vi "host_main.vi"() -> ()   [LabVIEW 2023]
uses:
  JSON Command.ctl
  Action.ctl
  <vilib>/rvi/interface/nirviOpenFPGA/nirviOpenFPGA.xnode
  <vilib>/rvi/interface/nirviReadWriteControl/nirviReadWriteControl.xnode
  <vilib>/rvi/interface/nirviMethod/nirviMethod.xnode
  <vilib>/FPGAPlugInAG/Dynamic/niLvFpga_ConfigureFifo_Dynamic.vi
  <vilib>/rvi/errors/niLvFpgaMergeErrorWithErrorCode.vi
  <vilib>/FPGAPlugInAG/Dynamic/niLvFpga_Run_Dynamic.vi
  <vilib>/FPGAPlugInAG/Dynamic/niLvFpga_WriteFifo_Dynamic.vi
  NiFpgaLv.dll
  <vilib>/Utility/error.llb/Error Cluster From Error Code.vi
  <vilib>/rvi/interface/Simulation/niFpgaSimulationCallBeginRW.vi
  <vilib>/rvi/errors/niLvFpgaAdjustHostInterfaceError.vi
  <vilib>/rvi/interface/nirviCloseFPGA/nirviCloseFPGA.xnode
  <vilib>/FPGAPlugInAG/Dynamic/niLvFpga_ReadFifo_Dynamic.vi
  <vilib>/FPGAPlugInAG/Dynamic/niLvFpga_StopFifo_Dynamic.vi
  LabView workspace/CoboltLaserDriver.lvlib
  <vilib>/FPGAPlugInAG/Dynamic/niLvFpga_Close_Dynamic.vi
  FPGA Bitfiles/cryosimcontrolsy_FPGATarget_targetmainmem_OolXwFFypuY.lvbitx
  target_main_mem.vi
  <vilib>/FPGAPlugInAG/cRIO-9048/niLvFpga_Open_cRIO-9048.vi
  <vilib>/rvi/interface/common/dynamic/niFpgaDynamicAddResources.vi
panel:
  in  "Stop VI":bool
  out "FPGA VI Reference Out":refnum<k20>
  out "Abort":bool
  out "remote port":u16
  out "remote address":string
  in  "Send PORT":u16=7704
  out "From Client:":string
  out "RAW JSON":T1
  out "ACK sent":string
  in  "FPGA Status Update Loop Time (uSec)":u32=1000
  out "UDP Sent":string
  in  "Event":string
  in  "FPGA Status":string
  in  "Receive PORT":u16=7705
  in  "UDP Address (IP)":string="172.22.11.1"
  out "Digitals":u8
  out "Laser Response OK":bool=TRUE
  out "488 Blue Toggle":bool
  out "532 Red Toggle":bool
  out "638 Green Toggle":bool
  in  "Analogue Line 5":u32=20
  in  "Analogue Line 4":u32=20
  in  "Analogue Line 3":u32=20
  out "Analogue Line 2":u8
  out "Analogue Line 1":u8
  out "Analogue Line 0":u8
  out "Tick Ref":u32
  out "Addr Digitals":u32
  out "repDuration (ms)":u64
  out "numReps":u64
  out "From sendStartStopIndexes":u64[](array[numeric])
  out "Addr Analogue 1":u32
  out "Addr Analogue 2":u32
  out "Addr Analogue 0":u32
  in  "Digitals Action Table":T2[](array[typedef])
  in  "Analogue 2 Action Table":T2[](array[typedef])
  in  "Analogue 1 Action Table":T2[](array[typedef])
  in  "Analogue 0 Action Table":T2[](array[typedef])
  # "TCP Communication"
  # "UDP Communication"
  # "FPGA: Angle, Phase, and Color"
  # "FPGA: Laser On/Off and Power Control"
  # "Action Tables & Experiment Logging"
  # "Experiment Execution Trace"
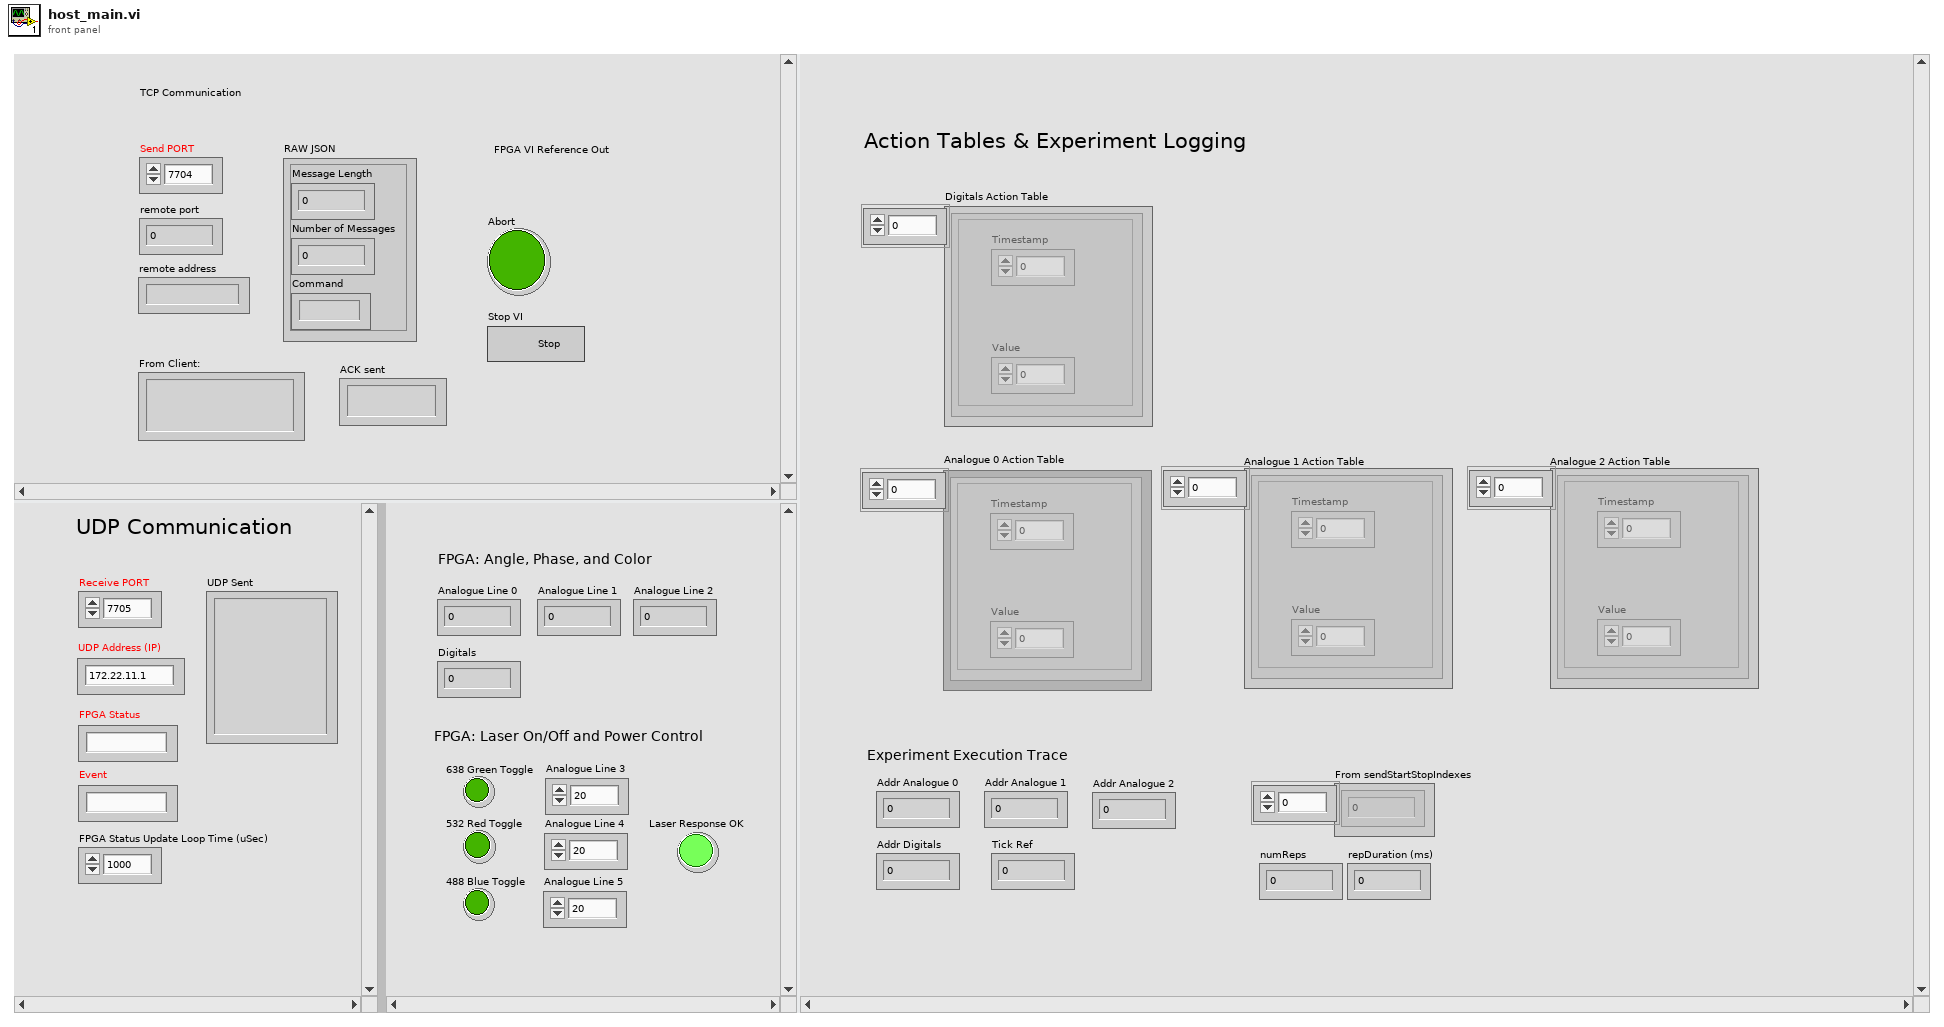
[diagram p1: front panel]
types:
  T1 = typedef "JSON Command.ctl" = cluster{"Message Length":i32, "Number of Messages":i32, "Command":string}
  T2 = typedef "Action.ctl" = cluster{"Timestamp":u32, "Value":u32}
  T3 = cluster{"Digital 0":bool, "Digital 1":bool, "Digital 2":bool}
  T4 = cluster{"Digitals":u8, "Analogue 0":u8, "Analogue 1":u8, "Event":string, "Analogue 2":u8, "Analogue 3":u32, "Analogue 4":u32, "Analogue 5":u32}
  T5 = enum16{"Standard", "Buffered", "CRLF", "Immediate"}
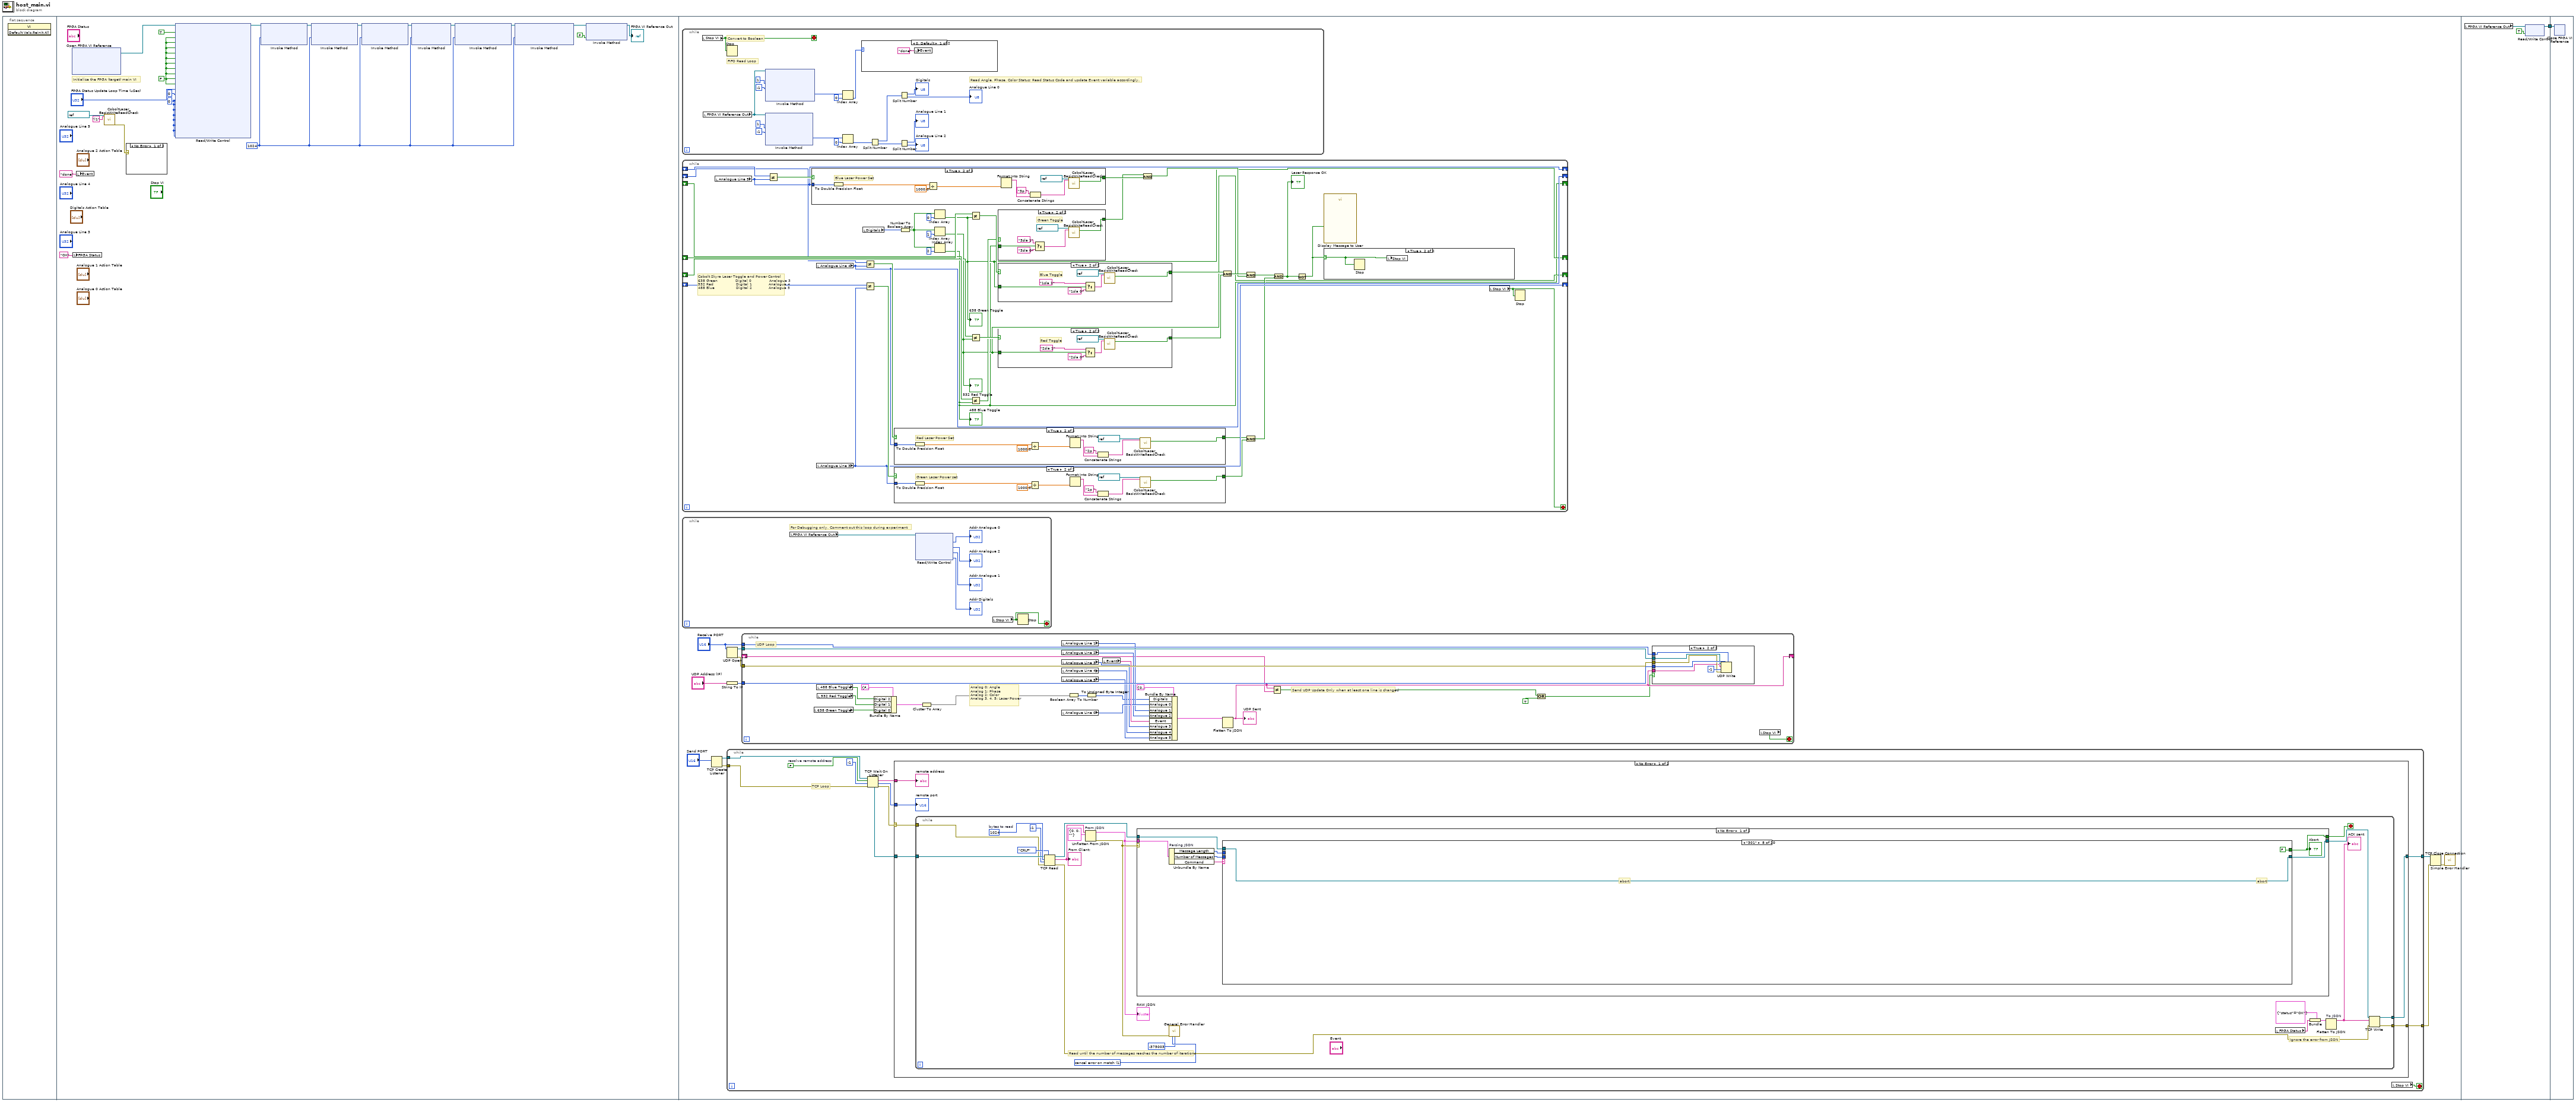
[diagram p0: block diagram]
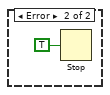
[diagram p2: hidden frame]
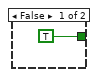
[diagram p4: hidden frame]
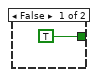
[diagram p5: hidden frame]
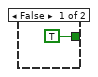
[diagram p6: hidden frame]
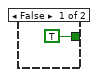
[diagram p7: hidden frame]
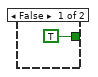
[diagram p8: hidden frame]
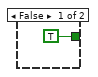
[diagram p9: hidden frame]
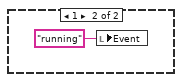
[diagram p10: hidden frame]
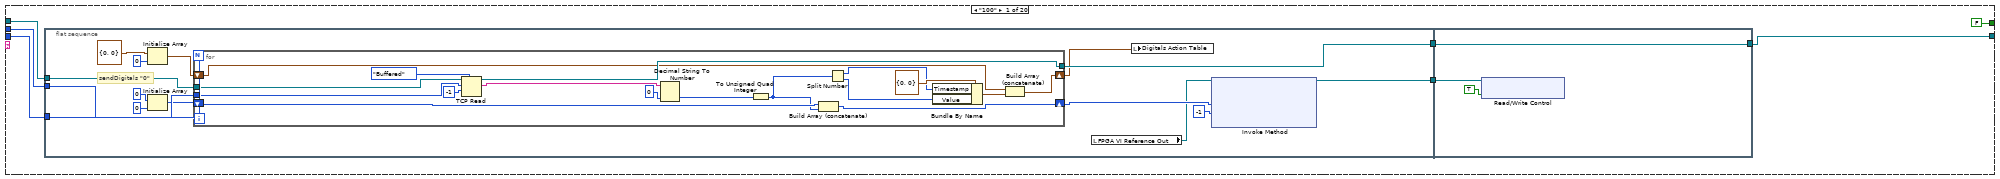
[diagram p12: hidden frame]
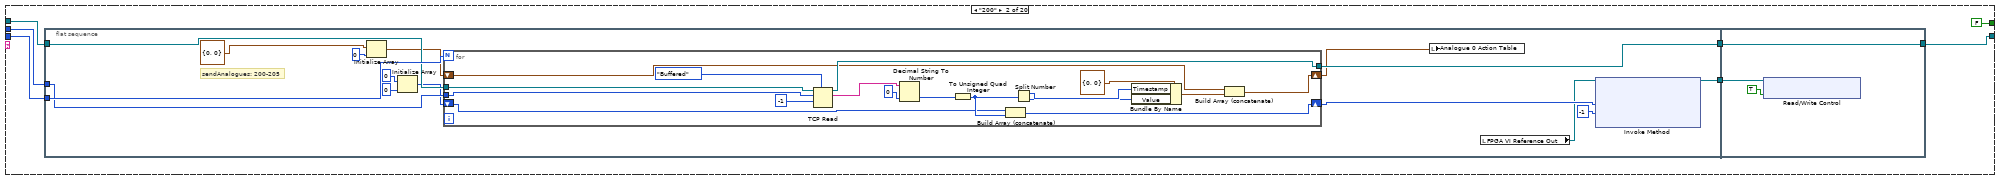
[diagram p13: hidden frame]
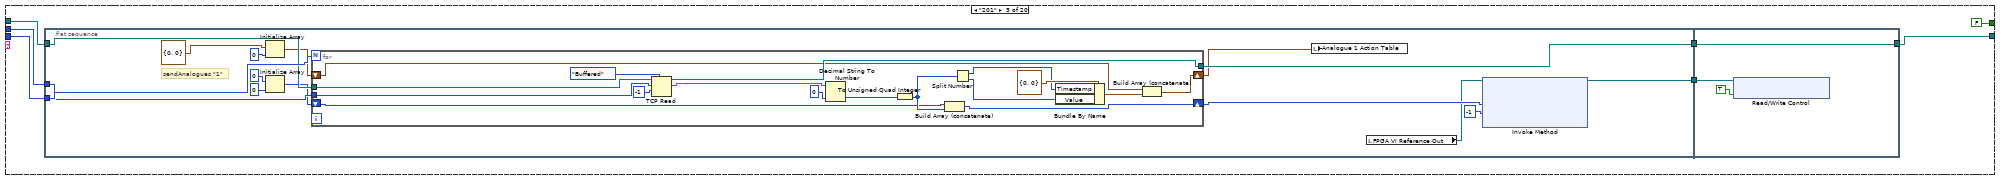
[diagram p14: hidden frame]
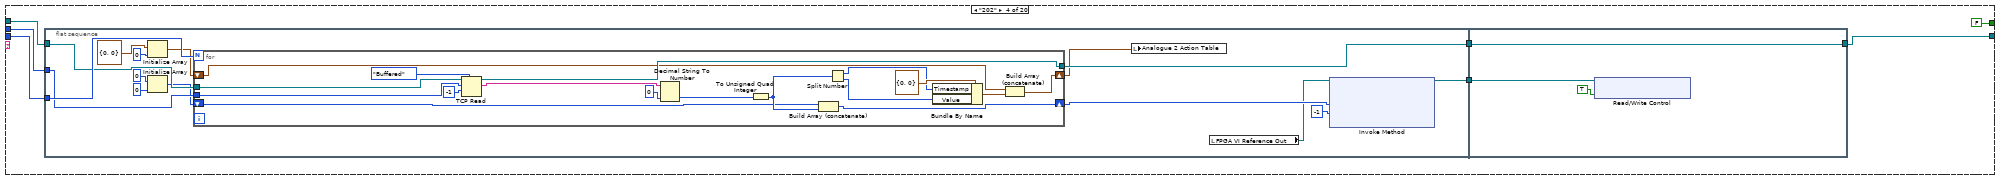
[diagram p15: hidden frame]
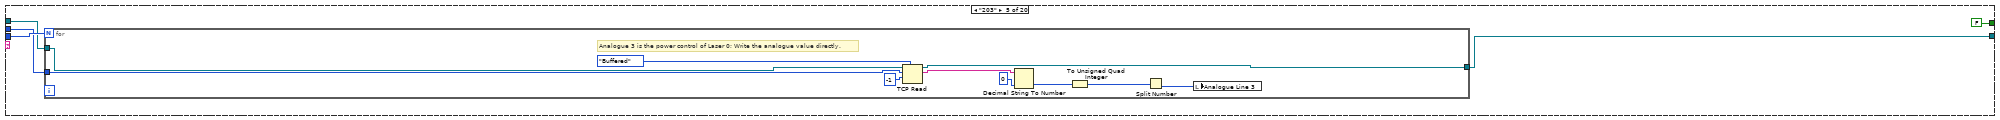
[diagram p16: hidden frame]
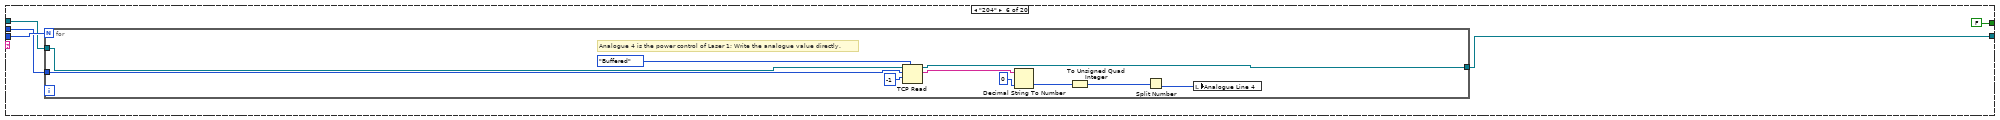
[diagram p17: hidden frame]
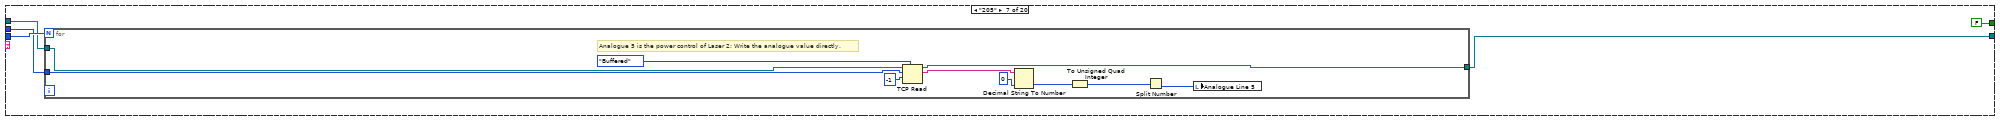
[diagram p18: hidden frame]
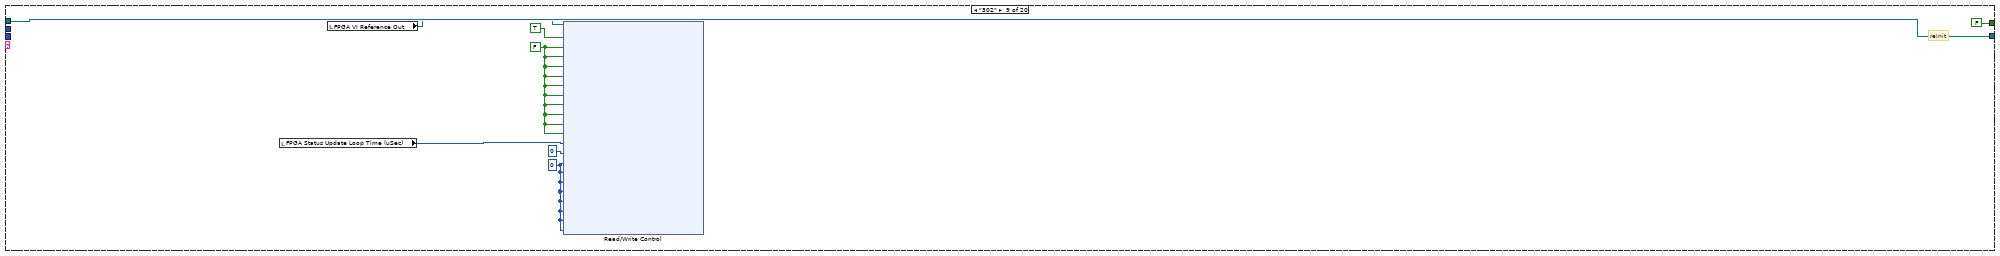
[diagram p19: hidden frame]
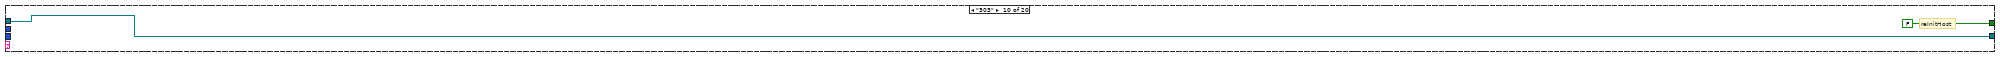
[diagram p20: hidden frame]
diagram:
  n1 = flat-sequence {
    tunnel: [w633] -> w1
    tunnel: w1 -> [w635]
    frame #0 {
      n2 = invoke class="VI" method="Default Vals.Reinit All"() -> ()  [unwired: 3 in, 3 out]
    }
    frame #1 {
      w5 = u32 0 ("Addr Analogue 0")
      w4 = u32 1024 ("Requested Depth")
      w2 = FALSE ("Action Abort")
      # "Initialize the FPGA (target) main VI"
      n3 = xnode "Open FPGA VI Reference"() -> ("FPGA VI Reference Out"=w11:refnum<k20>)  [unwired: 2 in, 1 out]
      n4 = local write "FPGA Status"("OK") -> ()
      n5 = local write "Event"("done") -> ()
      n6 = call "CoboltLaser_BasicWriteReadCheck.vi"("ComPort"=refnum<visa-resource-name> "COM4", "Command"="l1") -> ("error out"=w8:errorcluster)  [unwired: 22 in, 3 out]
      n7 = case shown="No Error" w8 {
        frame No Error {
        }
        frame Error {
          n8 = Stop(stop? (T)=TRUE) -> ()
        }
      }
      n9 = xnode "Read/Write Control"("FPGA VI Reference In"=w11, "FPGA Tick Reset"=TRUE, "Abort"=w2, "Load Actions Analogue 0"=w2, "Load Actions Analogue 1"=w2, "Load Actions Analogue 2"=w2, "Load Actions Digitals"=w2, "Flush FIFO"=w2, "Trigger Experiment"=w2, "Set Analogue 0"=w2, "Set Analogue 1"=w2, "Set Analogue 2"=w2, "FPGA Status Update Loop Time (uSec)"="FPGA Status Update Loop Time (uSec)", "Status Code"=u8 0, "Addr Analogue 0"=w5, "Addr Analogue 1"=w5, "Addr Analogue 2"=w5, "Num of Actions Analogue 0"=w5, "Num of Actions Analogue 1"=w5, "Num of Actions Analogue 2"=w5, "Num of Actions Digitals"=w5, "Digitals"=w5) -> ("FPGA VI Reference Out"=w7:refnum<k20>)  [unwired: 1 in, 1 out]
      n10 = xnode "Invoke Method"("FPGA VI Reference In"=w7, "Requested Depth"=w4) -> ("FPGA VI Reference Out"=w21:refnum<k20>)  [unwired: 1 in, 2 out]
      n11 = xnode "Invoke Method"("FPGA VI Reference In"=w21, "Requested Depth"=w4) -> ("FPGA VI Reference Out"=w12:refnum<k20>)  [unwired: 1 in, 2 out]
      n12 = xnode "Invoke Method"("FPGA VI Reference In"=w12, "Requested Depth"=w4) -> ("FPGA VI Reference Out"=w20:refnum<k20>)  [unwired: 1 in, 2 out]
      n13 = xnode "Invoke Method"("FPGA VI Reference In"=w20, "Requested Depth"=w4) -> ("FPGA VI Reference Out"=w19:refnum<k20>)  [unwired: 1 in, 2 out]
      n14 = xnode "Invoke Method"("FPGA VI Reference In"=w19, "Requested Depth"=w4) -> ("FPGA VI Reference Out"=w18:refnum<k20>)  [unwired: 1 in, 2 out]
      n15 = xnode "Invoke Method"("FPGA VI Reference In"=w18, "Requested Depth"=w4) -> ("FPGA VI Reference Out"=w6:refnum<k20>)  [unwired: 1 in, 2 out]
      n16 = xnode "Invoke Method"("FPGA VI Reference In"=w6, "Wait Until Done (F)"=FALSE) -> ("FPGA VI Reference Out"=→"FPGA VI Reference Out":refnum<k20>)  [unwired: 1 in, 1 out]
    }
    frame #2 {
      n17 = while {
        stop <- w130 stop-if-true
        # "Read Angle, Phase, Color Status; Read Status Code and update Event variable accordingly."
        # "FIFO Read Loop"
        # "Convert to Boolean"
        n18 = local read "Stop VI"() -> (w130:bool)
        n19 = local read "FPGA VI Reference Out"() -> (w131:refnum<k20>)
        n20 = Stop(stop? (T)=w130) -> ()
        n21 = xnode "Invoke Method"("FPGA VI Reference In"=w131, "Number of Elements"=u32 1, "Timeout (ms)"=-1) -> ("Data"=w135:u8[])  [unwired: 1 in, 3 out]
        n22 = xnode "Invoke Method"("FPGA VI Reference In"=w131, "Number of Elements"=u32 1, "Timeout (ms)"=-1) -> ("Data"=w144:u32[])  [unwired: 1 in, 3 out]
        n23 = Index Array(array=w135, index=0) -> (element=w136:u8)
        n24 = Index Array(array=w144, index=0) -> (element=w142:u32)
        n25 = case shown="0, Default" w136 {
          frame 0, Default {
            n26 = local write "Event"("done") -> ()
          }
          frame 1 {
            n27 = local write "Event"("running") -> ()
          }
        }
        n28 = Split Number(x=w142) -> (hi(x)=w141:u16, lo(x)=w140:u16)
        n29 = Split Number(x=w141) -> (hi(x)=→"Digitals":u8, lo(x)=→"Analogue Line 0":u8)
        n30 = Split Number(x=w140) -> (hi(x)=→"Analogue Line 1":u8, lo(x)=→"Analogue Line 2":u8)
      }
      n31 = while {
        shift-right: [w38] -> _
        shift-left: _ -> [w70]
        shift-right: [w36] -> _
        shift-left: _ -> [w65]
        shift-right: [w35] -> _
        shift-left: _ -> [w66]
        shift-right: [w58] -> _
        shift-left: _ -> [w61]
        shift-right: [w57] -> _
        shift-left: _ -> [w60]
        shift-right: [w56] -> _
        shift-left: _ -> [w59]
        stop <- w45 stop-if-true
        # "Cobolt Skyra Laser Toggle and Power Control\n638 Green               Digital 0               Analogue 3\n532 Red                   Digital 1              Analogue 4\n488 Blue                  Digital 2              Analogue 5"
        n32 = local read "Analogue Line 5"() -> (w58:u32)
        n33 = Not Equal?(x=w61, y=w58) -> (x != y?=w64:bool)
        n34 = case shown="True" w64 {
          tunnel: w58 -> [_ w96]
          tunnel: [TRUE w93] -> w53
          frame False {
          }
          frame True {
            # "Blue Laser Power Set"
            n35 = To Double Precision Float(number=w96) -> (double precision float=w97:dbl)
            n36 = Divide(x=w97, y=1000.0) -> (x/y=w101:dbl)
            n37 = Format Into String(w101) -> (resulting string=w100:string)  [unwired: 3 in, 1 out]
            n38 = Concatenate Strings("3p " ("string"), w100) -> (w95:string)
            n39 = call "CoboltLaser_BasicWriteReadCheck.vi"("ComPort"=refnum<visa-resource-name> "COM4", "Command"=w95) -> ("ResponseOK"=w93:bool)  [unwired: 22 in, 3 out]
          }
        }
        n40 = local read "Analogue Line 4"() -> (w57:u32)
        n41 = local read "Analogue Line 3"() -> (w56:u32)
        n42 = local read "Digitals"() -> (w37:u8)
        n43 = Not Equal?(x=w60, y=w57) -> (x != y?=w63:bool)
        n44 = Not Equal?(x=w59, y=w56) -> (x != y?=w62:bool)
        n45 = case shown="True" w63 {
          tunnel: w57 -> [_ w86]
          tunnel: [TRUE w84] -> w51
          frame False {
          }
          frame True {
            # "Red Laser Power Set"
            n46 = To Double Precision Float(number=w86) -> (double precision float=w87:dbl)
            n47 = Divide(x=w87, y=1000.0) -> (x/y=w91:dbl)
            n48 = Format Into String(w91) -> (resulting string=w90:string)  [unwired: 3 in, 1 out]
            n49 = Concatenate Strings("2p " ("string"), w90) -> (w83:string)
            n50 = call "CoboltLaser_BasicWriteReadCheck.vi"("ComPort"=refnum<visa-resource-name> "COM4", "Command"=w83) -> ("ResponseOK"=w84:bool)  [unwired: 22 in, 3 out]
          }
        }
        n51 = case shown="True" w62 {
          tunnel: w56 -> [_ w76]
          tunnel: [TRUE w74] -> w50
          frame False {
          }
          frame True {
            # "Green Laser Power set"
            n52 = To Double Precision Float(number=w76) -> (double precision float=w77:dbl)
            n53 = Divide(x=w77, y=1000.0) -> (x/y=w81:dbl)
            n54 = Format Into String(w81) -> (resulting string=w80:string)  [unwired: 3 in, 1 out]
            n55 = Concatenate Strings("1p " ("string"), w80) -> (w73:string)
            n56 = call "CoboltLaser_BasicWriteReadCheck.vi"("ComPort"=refnum<visa-resource-name> "COM4", "Command"=w73) -> ("ResponseOK"=w74:bool)  [unwired: 22 in, 3 out]
          }
        }
        n57 = Number To Boolean Array(number=w37) -> (Boolean array=w39:bool[])
        n58 = Index Array(array=w39, index=0) -> (element=w38:bool)
        "638 Green Toggle" <- w38
        n59 = Index Array(array=w39, index=1) -> (element=w36:bool)
        "532 Red Toggle" <- w36
        n60 = Index Array(array=w39, index=2) -> (element=w35:bool)
        "488 Blue Toggle" <- w35
        n61 = Not Equal?(x=w70, y=w38) -> (x != y?=w69:bool)
        n62 = Not Equal?(x=w65, y=w36) -> (x != y?=w68:bool)
        n63 = Not Equal?(x=w66, y=w35) -> (x != y?=w67:bool)
        n64 = case shown="True" w67 {
          tunnel: w35 -> [_ w105]
          tunnel: [TRUE w103] -> w52
          frame False {
          }
          frame True {
            # "Green Toggle"
            n65 = Select(t="3sla 1", s=w105, f="3sla 0") -> (s? t:f=w104:string)
            n66 = call "CoboltLaser_BasicWriteReadCheck.vi"("ComPort"=refnum<visa-resource-name> "COM4", "Command"=w104) -> ("ResponseOK"=w103:bool)  [unwired: 22 in, 3 out]
          }
        }
        n67 = case shown="True" w69 {
          tunnel: w38 -> [_ w120]
          tunnel: [TRUE w117] -> w55
          frame False {
          }
          frame True {
            # "Blue Toggle"
            n68 = Select(t="1sla 1", s=w120, f="1sla 0") -> (s? t:f=w118:string)
            n69 = call "CoboltLaser_BasicWriteReadCheck.vi"("ComPort"=refnum<visa-resource-name> "COM4", "Command"=w118) -> ("ResponseOK"=w117:bool)  [unwired: 22 in, 3 out]
          }
        }
        n70 = case shown="True" w68 {
          tunnel: w36 -> [_ w111]
          tunnel: [TRUE w110] -> w54
          frame False {
          }
          frame True {
            # "Red Toggle"
            n71 = Select(t="2sla 1", s=w111, f="2sla 0") -> (s? t:f=w112:string)
            n72 = call "CoboltLaser_BasicWriteReadCheck.vi"("ComPort"=refnum<visa-resource-name> "COM4", "Command"=w112) -> ("ResponseOK"=w110:bool)  [unwired: 22 in, 3 out]
          }
        }
        n73 = And(x=w52, y=w53) -> (x .and. y?=w48:bool)
        n74 = And(x=w55, y=w54) -> (x .and. y?=w49:bool)
        n75 = And(x=w49, y=w48) -> (x .and. y?=w46:bool)
        n76 = And(x=w51, y=w50) -> (x .and. y?=w47:bool)
        n77 = And(x=w46, y=w47) -> (x .and. y?=w44:bool)
        "Laser Response OK" <- w44
        n78 = Not(x=w44) -> (.not. x?=w43:bool)
        n79 = call "Display Message to User"("Enable"=w43) -> ()  [unwired: 9 in, 2 out]
        n80 = case shown="True" w43 {
          selector: w43 -> [_ w71]
          frame False {
          }
          frame True {
            n81 = Stop(stop? (T)=w71) -> ()
            n82 = local write "Stop VI"(w71) -> ()
          }
        }
        n83 = local read "Stop VI"() -> (w45:bool)
        n84 = Stop(stop? (T)=w45) -> ()
      }
      n85 = while {
        stop <- w124 stop-if-true
        # "For Debugging only. Comment out this loop during experiment"
        n86 = local read "FPGA VI Reference Out"() -> (w125:refnum<k20>)
        n87 = xnode "Read/Write Control"("FPGA VI Reference In"=w125) -> ("Addr Analogue 0"=→"Addr Analogue 0":u32, "Addr Analogue 2"=→"Addr Analogue 2":u32, "Addr Analogue 1"=→"Addr Analogue 1":u32, "Addr Digitals"=→"Addr Digitals":u32)  [unwired: 1 in, 2 out]
        n88 = local read "Stop VI"() -> (w124:bool)
        n89 = Stop(stop? (T)=w124) -> ()
      }
      n90 = TCP Create Listener(10:"Send PORT") -> (0:w32:errorcluster, 3:w31:refnum<k5>)  [unwired: 4 in, 1 out]
      n91 = UDP Open(11:"Receive PORT") -> (port=w26:refnum<k16>, 0:w28:errorcluster)  [unwired: 4 in, 1 out]
      n92 = String To IP(1:"UDP Address (IP)") -> (0:w25:u32)
      n93 = while {
        tunnel: w31 -> [w192]
        tunnel: w32 -> [w191]
        tunnel: [w190] -> w33
        tunnel: [w189] -> w34
        stop <- w182 stop-if-true
        w186 = FALSE  # resolve remote address
        # "TCP Loop"
        n94 = TCP Wait On Listener(8:w191, 9:-1 ("timeout ms (wait forever: -1)"), 10:w186, 11:w192) -> (0:w187:errorcluster, 1:w184:u16, 2:w185:string, 4:w183:refnum<k5>)  [unwired: 1 out]
        n95 = case shown="No Error" w187 {
          selector: w187 -> [w195 w630]
          tunnel: w183 -> [w198 w631]
          tunnel: [w197 w630] -> w190
          tunnel: [w196 w631] -> w189
          tunnel: w185 -> [w193 _]
          tunnel: w184 -> [w194 _]
          frame No Error {
            n96 = while {
              tunnel: w195 -> [w209]
              tunnel: [w211] -> w197
              tunnel: w198 -> [w212]
              tunnel: [w210] -> w196
              stop <- w203 stop-if-true
              w207 = 1 items=["no exception", "cancel error on match", "set error on match"] ("[exception action] (none:0)")
              w218 = 1024  # bytes to read
              # "Ignore the error from JSON"
              # "Read until the number of messages reaches the number of iterations"
              n97 = TCP Read(connection ID=w212, bytes to read=w218, error in (no error)=w209, 7:T5."CRLF" ("mode (standard)"), 9:-1 ("timeout ms (25000)")) -> (connection ID out=w201:refnum<k5>, data out=w215:string, error out=w219:errorcluster)
              "From Client:" <- w215
              n98 = Unflatten From JSON "From JSON"(JSON string=w215, type and defaults=T1 {"Message Length"=0, "Number of Messages"=0, "Command"=""} ("JSON Command")) -> (value=w204:T1, error out=w205:errorcluster)  [unwired: 5 in]
              "RAW JSON" <- w204
              n99 = case shown="No Error" w205 {
                tunnel: w204 -> [w226 _]
                tunnel: [w224 TRUE] -> w203
                tunnel: w201 -> [w222 w628]
                tunnel: [w221 w628] -> w200
                frame No Error {
                  n100 = Unbundle By Name "Parsing JSON"(w226) -> ("Message Length"=w220:i32, "Number of Messages"=w223:i32, "Command"=w225:string)
                  n101 = case shown="\"301\"" w225 {
                    tunnel: [FALSE FALSE FALSE FALSE FALSE FALSE FALSE FALSE FALSE FALSE FALSE FALSE FALSE FALSE FALSE FALSE FALSE FALSE FALSE TRUE] -> w224
                    tunnel: w223 -> [w232 w274 w317 w358 w398 w413 w428 _ _ _ _ _ w477 w500 _ _ _ _ _ _]
                    tunnel: w222 -> [w231 w273 w315 w357 w397 w412 w427 w440 w448 w450 w453 w469 w478 w502 w516 w535 w557 w572 w624 w627]
                    tunnel: [w230 w272 w314 w355 w395 w410 w425 w440 w448 w450 w453 w469 w471 w491 w516 w535 w556 w563 w624 w627] -> w221
                    tunnel: w220 -> [w229 w271 w313 w356 w396 w411 w426 _ _ _ _ _ w476 w501 _ _ w554 w568 _ _]
                    frame "100" {
                      n102 = flat-sequence {
                        tunnel: w232 -> [w248]
                        tunnel: w231 -> [w247]
                        tunnel: w229 -> [w245]
                        tunnel: [w246] -> w228
                        tunnel: [w234] -> w227
                        tunnel: [w268] -> w230
                        tunnel: w228 -> [w268]
                        tunnel: w227 -> [w267]
                        frame #0 {
                          # "sendDigitals \"0\""
                          n103 = Initialize Array(T2 {"Timestamp"=0, "Value"=0} ("Action"), 0 ("dimension size")) -> (w240:T2[])
                          n104 = Initialize Array(u64 0 ("element"), 0 ("dimension size")) -> (w239:u64[])
                          n105 = for {
                            N: w248 -> [_]
                            tunnel: w247 -> [w264]
                            tunnel: [w263] -> w246
                            tunnel: w245 -> [w262]
                            shift-right: [w250] -> w237
                            shift-left: w239 -> [w252]
                            shift-right: [w253] -> w238
                            shift-left: w240 -> [w255]
                            n106 = TCP Read(connection ID=w264, bytes to read=w262, 7:T5."Buffered" ("mode (standard)"), 9:-1 ("timeout ms (25000)")) -> (connection ID out=w263:refnum<k5>, data out=w259:string)  [unwired: 1 in, 1 out]
                            n107 = Decimal String To Number(string=w259, default (0L)=u64 0 ("default (0 I32)")) -> (number=w260:u64)  [unwired: 1 in, 1 out]
                            n108 = To Unsigned Quad Integer(1:w260) -> (0:w251:u64)
                            n109 = Build Array (concatenate)(w252, w251) -> (w250:u64[])
                            n110 = Split Number(x=w251) -> (hi(x)=w257:u32, lo(x)=w256:u32)
                            n111 = Bundle By Name(cluster=T2 {"Timestamp"=0, "Value"=0} ("Action"), "Timestamp"=w257, "Value"=w256) -> (w254:T2)
                            n112 = Build Array (concatenate)(w255, w254) -> (w253:T2[])
                          }
                          n113 = local read "FPGA VI Reference Out"() -> (w235:refnum<k20>)
                          n114 = local write "Digitals Action Table"(w238) -> ()
                          n115 = xnode "Invoke Method"("FPGA VI Reference In"=w235, "Data"=w237, "Timeout (ms)"=-1) -> ("FPGA VI Reference Out"=w234:refnum<k20>)  [unwired: 1 in, 2 out]
                        }
                        frame #1 {
                          n116 = xnode "Read/Write Control"("FPGA VI Reference In"=w267, "Load Actions Digitals"=TRUE ("Load Actions")) -> ()  [unwired: 1 in, 2 out]
                        }
                      }
                    }
                    frame "200" {
                      n117 = flat-sequence {
                        tunnel: w274 -> [w290]
                        tunnel: w273 -> [w289]
                        tunnel: w271 -> [w287]
                        tunnel: [w288] -> w270
                        tunnel: [w276] -> w269
                        tunnel: [w310] -> w272
                        tunnel: w270 -> [w310]
                        tunnel: w269 -> [w309]
                        frame #0 {
                          # "sendAnalogues: 200-205"
                          n118 = Initialize Array(T2 {"Timestamp"=0, "Value"=0} ("Action"), 0 ("dimension size")) -> (w284:T2[])
                          n119 = Initialize Array(u64 0 ("element"), 0 ("dimension size")) -> (w280:u64[])
                          n120 = for {
                            N: w290 -> [_]
                            tunnel: w289 -> [w306]
                            tunnel: [w304] -> w288
                            tunnel: w287 -> [w303]
                            shift-right: [w294] -> w283
                            shift-left: w284 -> [w299]
                            shift-right: [w291] -> w279
                            shift-left: w280 -> [w292]
                            n121 = TCP Read(connection ID=w306, bytes to read=w303, 7:T5."Buffered" ("mode (standard)"), 9:-1 ("timeout ms (25000)")) -> (connection ID out=w304:refnum<k5>, data out=w301:string)  [unwired: 1 in, 1 out]
                            n122 = Decimal String To Number(string=w301, default (0L)=u64 0) -> (number=w302:u64)  [unwired: 1 in, 1 out]
                            n123 = To Unsigned Quad Integer(1:w302) -> (0:w293:u64)
                            n124 = Build Array (concatenate)(w292, w293) -> (w291:u64[])
                            n125 = Split Number(x=w293) -> (hi(x)=w297:u32, lo(x)=w296:u32)
                            n126 = Bundle By Name(cluster=T2 {"Timestamp"=0, "Value"=0} ("Action"), "Timestamp"=w297, "Value"=w296) -> (w295:T2)
                            n127 = Build Array (concatenate)(w299, w295) -> (w294:T2[])
                          }
                          n128 = local write "Analogue 0 Action Table"(w283) -> ()
                          n129 = local read "FPGA VI Reference Out"() -> (w277:refnum<k20>)
                          n130 = xnode "Invoke Method"("FPGA VI Reference In"=w277, "Data"=w279, "Timeout (ms)"=-1) -> ("FPGA VI Reference Out"=w276:refnum<k20>)  [unwired: 1 in, 2 out]
                        }
                        frame #1 {
                          n131 = xnode "Read/Write Control"("FPGA VI Reference In"=w309, "Load Actions Analogue 0"=TRUE ("Load Actions")) -> ()  [unwired: 1 in, 2 out]
                        }
                      }
                    }
                    frame "201" {
                      n132 = flat-sequence {
                        tunnel: w317 -> [w332]
                        tunnel: w315 -> [w331]
                        tunnel: w313 -> [w329]
                        tunnel: [w330] -> w312
                        tunnel: [w318] -> w311
                        tunnel: [w352] -> w314
                        tunnel: w312 -> [w352]
                        tunnel: w311 -> [w351]
                        frame #0 {
                          # "sendAnalogues \"1\""
                          n133 = Initialize Array(T2 {"Timestamp"=0, "Value"=0} ("Action"), 0 ("dimension size")) -> (w326:T2[])
                          n134 = Initialize Array(u64 0, 0 ("dimension size")) -> (w321:u64[])
                          n135 = for {
                            N: w332 -> [_]
                            tunnel: w331 -> [w349]
                            tunnel: [w348] -> w330
                            tunnel: w329 -> [w347]
                            shift-right: [w338] -> w324
                            shift-left: w326 -> [w339]
                            shift-right: [w335] -> w320
                            shift-left: w321 -> [w336]
                            n136 = TCP Read(connection ID=w349, bytes to read=w347, 7:T5."Buffered" ("mode (standard)"), 9:-1 ("timeout ms (25000)")) -> (connection ID out=w348:refnum<k5>, data out=w344:string)  [unwired: 1 in, 1 out]
                            n137 = Decimal String To Number(string=w344, default (0L)=u64 0 ("default (0 I32)")) -> (number=w343:u64)  [unwired: 1 in, 1 out]
                            n138 = To Unsigned Quad Integer(1:w343) -> (0:w337:u64)
                            n139 = Build Array (concatenate)(w336, w337) -> (w335:u64[])
                            n140 = Split Number(x=w337) -> (hi(x)=w334:u32, lo(x)=w342:u32)
                            n141 = Bundle By Name(cluster=T2 {"Timestamp"=0, "Value"=0} ("Action"), "Timestamp"=w334, "Value"=w342) -> (w340:T2)
                            n142 = Build Array (concatenate)(w339, w340) -> (w338:T2[])
                          }
                          n143 = local write "Analogue 1 Action Table"(w324) -> ()
                          n144 = local read "FPGA VI Reference Out"() -> (w319:refnum<k20>)
                          n145 = xnode "Invoke Method"("FPGA VI Reference In"=w319, "Data"=w320, "Timeout (ms)"=-1) -> ("FPGA VI Reference Out"=w318:refnum<k20>)  [unwired: 1 in, 2 out]
                        }
                        frame #1 {
                          n146 = xnode "Read/Write Control"("FPGA VI Reference In"=w351, "Load Actions Analogue 1"=TRUE ("Load Actions")) -> ()  [unwired: 1 in, 2 out]
                        }
                      }
                    }
                    frame "202" {
                      n147 = flat-sequence {
                        tunnel: w358 -> [w374]
                        tunnel: w357 -> [w369]
                        tunnel: w356 -> [w368]
                        tunnel: [w367] -> w354
                        tunnel: [w361] -> w353
                        tunnel: [w394] -> w355
                        tunnel: w354 -> [w394]
                        tunnel: w353 -> [w393]
                        frame #0 {
                          n148 = Initialize Array(T2 {"Timestamp"=0, "Value"=0} ("Action"), 0 ("dimension size")) -> (w366:T2[])
                          n149 = Initialize Array(u64 0 ("element"), 0 ("dimension size")) -> (w364:u64[])
                          n150 = for {
                            N: w374 -> [_]
                            tunnel: w369 -> [w390]
                            tunnel: w368 -> [w389]
                            tunnel: [w386] -> w367
                            shift-right: [w379] -> w365
                            shift-left: w366 -> [w380]
                            shift-right: [w376] -> w363
                            shift-left: w364 -> [w377]
                            n151 = TCP Read(connection ID=w390, bytes to read=w389, 7:T5."Buffered" ("mode (standard)"), 9:-1 ("timeout ms (25000)")) -> (connection ID out=w386:refnum<k5>, data out=w387:string)  [unwired: 1 in, 1 out]
                            n152 = Decimal String To Number(string=w387, default (0L)=u64 0 ("default (0 I32)")) -> (number=w385:u64)  [unwired: 1 in, 1 out]
                            n153 = To Unsigned Quad Integer(1:w385) -> (0:w378:u64)
                            n154 = Build Array (concatenate)(w377, w378) -> (w376:u64[])
                            n155 = Split Number(x=w378) -> (hi(x)=w383:u32, lo(x)=w382:u32)
                            n156 = Bundle By Name(cluster=T2 {"Timestamp"=0, "Value"=0} ("Action"), "Timestamp"=w383, "Value"=w382) -> (w381:T2)
                            n157 = Build Array (concatenate)(w380, w381) -> (w379:T2[])
                          }
                          n158 = local write "Analogue 2 Action Table"(w365) -> ()
                          n159 = local read "FPGA VI Reference Out"() -> (w360:refnum<k20>)
                          n160 = xnode "Invoke Method"("FPGA VI Reference In"=w360, "Data"=w363, "Timeout (ms)"=-1) -> ("FPGA VI Reference Out"=w361:refnum<k20>)  [unwired: 1 in, 2 out]
                        }
                        frame #1 {
                          n161 = xnode "Read/Write Control"("FPGA VI Reference In"=w393, "Load Actions Analogue 2"=TRUE ("Load Actions")) -> ()  [unwired: 1 in, 2 out]
                        }
                      }
                    }
                    frame "203" {
                      n162 = for {
                        N: w398 -> [_]
                        tunnel: w397 -> [w408]
                        tunnel: w396 -> [w407]
                        tunnel: [w404] -> w395
                        # "Analogue 3 is the power control of Laser 0; Write the analogue value directly."
                        n163 = TCP Read(connection ID=w408, bytes to read=w407, 7:T5."Buffered" ("mode (standard)"), 9:-1 ("timeout ms (25000)")) -> (connection ID out=w404:refnum<k5>, data out=w405:string)  [unwired: 1 in, 1 out]
                        n164 = Decimal String To Number(string=w405, default (0L)=u64 0 ("default (0 I32)")) -> (number=w403:u64)  [unwired: 1 in, 1 out]
                        n165 = To Unsigned Quad Integer(1:w403) -> (0:w402:u64)
                        n166 = Split Number(x=w402) -> (lo(x)=w400:u32)  [unwired: 1 out]
                        n167 = local write "Analogue Line 3"(w400) -> ()
                      }
                    }
                    frame "204" {
                      n168 = for {
                        N: w413 -> [_]
                        tunnel: w412 -> [w423]
                        tunnel: w411 -> [w422]
                        tunnel: [w419] -> w410
                        # "Analogue 4 is the power control of Laser 1; Write the analogue value directly."
                        n169 = TCP Read(connection ID=w423, bytes to read=w422, 7:T5."Buffered" ("mode (standard)"), 9:-1 ("timeout ms (25000)")) -> (connection ID out=w419:refnum<k5>, data out=w420:string)  [unwired: 1 in, 1 out]
                        n170 = Decimal String To Number(string=w420, default (0L)=u64 0 ("default (0 I32)")) -> (number=w418:u64)  [unwired: 1 in, 1 out]
                        n171 = To Unsigned Quad Integer(1:w418) -> (0:w417:u64)
                        n172 = Split Number(x=w417) -> (lo(x)=w415:u32)  [unwired: 1 out]
                        n173 = local write "Analogue Line 4"(w415) -> ()
                      }
                    }
                    frame "205" {
                      n174 = for {
                        N: w428 -> [_]
                        tunnel: w427 -> [w438]
                        tunnel: w426 -> [w437]
                        tunnel: [w434] -> w425
                        # "Analogue 5 is the power control of Laser 2; Write the analogue value directly."
                        n175 = TCP Read(connection ID=w438, bytes to read=w437, 7:T5."Buffered" ("mode (standard)"), 9:-1 ("timeout ms (25000)")) -> (connection ID out=w434:refnum<k5>, data out=w435:string)  [unwired: 1 in, 1 out]
                        n176 = Decimal String To Number(string=w435, default (0L)=u64 0 ("default (0 I32)")) -> (number=w433:u64)  [unwired: 1 in, 1 out]
                        n177 = To Unsigned Quad Integer(1:w433) -> (0:w432:u64)
                        n178 = Split Number(x=w432) -> (lo(x)=w430:u32)  [unwired: 1 out]
                        n179 = local write "Analogue Line 5"(w430) -> ()
                      }
                    }
                    frame "301" {
                      # "abort"
                      # "abort"
                    }
                    frame "302" {
                      w445 = u32 0 ("Addr Analogue 0")
                      w444 = FALSE ("Action Abort")
                      # "reInit"
                      n180 = local read "FPGA Status Update Loop Time (uSec)"() -> (w442:u32)
                      n181 = local read "FPGA VI Reference Out"() -> (w443:refnum<k20>)
                      n182 = xnode "Read/Write Control"("FPGA VI Reference In"=w443, "FPGA Tick Reset"=TRUE, "Abort"=w444, "Load Actions Analogue 0"=w444, "Load Actions Analogue 1"=w444, "Load Actions Analogue 2"=w444, "Load Actions Digitals"=w444, "Flush FIFO"=w444, "Trigger Experiment"=w444, "Set Analogue 0"=w444, "Set Analogue 1"=w444, "Set Analogue 2"=w444, "FPGA Status Update Loop Time (uSec)"=w442, "Status Code"=u8 0, "Addr Analogue 0"=w445, "Addr Analogue 1"=w445, "Addr Analogue 2"=w445, "Num of Actions Analogue 0"=w445, "Num of Actions Analogue 1"=w445, "Num of Actions Analogue 2"=w445, "Num of Actions Digitals"=w445, "Digitals"=w445) -> ()  [unwired: 1 in, 2 out]
                    }
                    frame "303" {
                      # "reInitHost"
                    }
                    frame "304" {
                      # "reInitFPGA"
                      n183 = flat-sequence {
                        tunnel: [w458] -> w452
                        tunnel: w452 -> [w465]
                        frame #0 {
                          w457 = u32 0 ("Addr Analogue 0")
                          w455 = FALSE ("Abort")
                          w456 = TRUE ("FPGA Tick Reset")
                          n184 = local read "FPGA VI Reference Out"() -> (w464:refnum<k20>)
                          n185 = xnode "Read/Write Control"("FPGA VI Reference In"=w464, "FPGA Tick Reset"=w456, "Flush FIFO"=w456, "Load Actions Analogue 0"=w455, "Load Actions Analogue 1"=w455, "Load Actions Analogue 2"=w455, "Load Actions Digitals"=w455, "Abort"=w455, "Set Analogue 0"=w455, "Set Analogue 1"=w455, "Set Analogue 2"=w455, "Trigger Experiment"=w455, "Status Code"=u8 0, "Addr Analogue 0"=w457, "Addr Analogue 1"=w457, "Addr Analogue 2"=w457, "Addr Digitals"=w457, "Num of Actions Digitals"=w457, "Num of Actions Analogue 0"=w457, "Num of Actions Analogue 1"=w457, "Num of Actions Analogue 2"=w457) -> ("FPGA VI Reference Out"=w459:refnum<k20>)  [unwired: 1 in, 1 out]
                          n186 = xnode "Invoke Method"("FPGA VI Reference In"=w459) -> ("FPGA VI Reference Out"=w462:refnum<k20>)  [unwired: 1 in, 1 out]
                          n187 = xnode "Invoke Method"("FPGA VI Reference In"=w462) -> ("FPGA VI Reference Out"=w461:refnum<k20>)  [unwired: 1 in, 1 out]
                          n188 = xnode "Invoke Method"("FPGA VI Reference In"=w461) -> ("FPGA VI Reference Out"=w460:refnum<k20>)  [unwired: 1 in, 1 out]
                          n189 = xnode "Invoke Method"("FPGA VI Reference In"=w460) -> ("FPGA VI Reference Out"=w458:refnum<k20>)  [unwired: 1 in, 1 out]
                        }
                        frame #1 {
                          n190 = while {
                            tunnel: w465 -> [w466]
                            stop <- w467 stop-if-true
                            n191 = xnode "Read/Write Control"("FPGA VI Reference In"=w466) -> ("Flush FIFO"=w468:bool)  [unwired: 1 in, 2 out]
                            n192 = Not(x=w468) -> (.not. x?=w467:bool)
                          }
                        }
                      }
                    }
                    frame "405" {
                      # "updateNrReps"
                    }
                    frame "406" {
                      # "sendStartStopIndexes"
                      n193 = Initialize Array(u64 0 ("element"), 0 ("dimension size")) -> (w473:u64[])
                      n194 = for {
                        N: w477 -> [_]
                        tunnel: w478 -> [w489]
                        tunnel: w476 -> [w488]
                        shift-right: [w481] -> w472
                        shift-left: w473 -> [w484]
                        tunnel: [w480] -> w471
                        n195 = TCP Read(connection ID=w489, bytes to read=w488, 7:T5."Buffered" ("mode (standard)"), 9:-1 ("timeout ms (25000)")) -> (connection ID out=w480:refnum<k5>, data out=w486:string)  [unwired: 1 in, 1 out]
                        n196 = Decimal String To Number(string=w486, default (0L)=u64 0 ("default (0 I32)")) -> (number=w483:u64)  [unwired: 1 in, 1 out]
                        n197 = To Unsigned Quad Integer(1:w483) -> (0:w482:u64)
                        n198 = Build Array (concatenate)(w484, w482) -> (w481:u64[])
                      }
                      "From sendStartStopIndexes" <- w472
                    }
                    frame "407" {
                      # "initProfile"
                      n199 = Initialize Array(u64 0 ("element"), 0 ("dimension size")) -> (w497:u64[])
                      n200 = for {
                        N: w500 -> [_]
                        tunnel: w502 -> [w513]
                        tunnel: w501 -> [w512]
                        shift-right: [w505] -> w496
                        shift-left: w497 -> [w507]
                        tunnel: [w504] -> w491
                        n201 = TCP Read(connection ID=w513, bytes to read=w512, 9:-1 ("timeout ms (25000)")) -> (connection ID out=w504:refnum<k5>, data out=w510:string)  [unwired: 2 in, 1 out]
                        n202 = Decimal String To Number(string=w510, default (0L)=u64 0 ("default (0 I32)")) -> (number=w508:u64)  [unwired: 1 in, 1 out]
                        n203 = To Unsigned Quad Integer(1:w508) -> (0:w506:u64)
                        n204 = Build Array (concatenate)(w507, w506) -> (w505:u64[])
                      }
                      n205 = Index Array(array=w496, index=1) -> (element=→"repDuration (ms)":u64)
                      n206 = Index Array(array=w496, index=0) -> (element=→"numReps":u64)
                    }
                    frame "408" {
                      # "triggerExperiment"
                      n207 = local read "FPGA VI Reference Out"() -> (w515:refnum<k20>)
                      n208 = flat-sequence {
                        tunnel: w515 -> [w518]
                        tunnel: [w520] -> w514
                        tunnel: w514 -> [w533]
                        frame #0 {
                          n209 = while {
                            tunnel: w518 -> [w529]
                            stop <- w528 stop-if-true
                            # "wait until all actions loaded"
                            n210 = xnode "Read/Write Control"("FPGA VI Reference In"=w529) -> ("Load Actions Analogue 0"=w524:bool, "Load Actions Analogue 1"=w523:bool, "Load Actions Analogue 2"=w522:bool, "Load Actions Analogue 2"=w521:bool)  [unwired: 1 in, 2 out]
                            n211 = Or(x=w524, y=w523) -> (x .or. y?=w526:bool)
                            n212 = Or(x=w522, y=w521) -> (x .or. y?=w525:bool)
                            n213 = Or(x=w526, y=w525) -> (x .or. y?=w527:bool)
                            n214 = Not(x=w527) -> (.not. x?=w528:bool)
                          }
                          n215 = xnode "Read/Write Control"("FPGA VI Reference In"=w518, "FPGA Tick Reset"=TRUE) -> ("FPGA VI Reference Out"=w520:refnum<k20>)  [unwired: 1 in, 1 out]
                        }
                        frame #1 {
                          n216 = xnode "Read/Write Control"("FPGA VI Reference In"=w533, "FPGA Tick Reset"=FALSE, "Trigger Experiment"=TRUE ("FPGA Tick Reset")) -> ("Tick Ref"=→"Tick Ref":u32)  [unwired: 1 in, 2 out]
                        }
                      }
                    }
                    frame "409" {
                      # "flushFIFOs"
                      n217 = flat-sequence {
                        tunnel: [w538] -> w534
                        tunnel: w534 -> [w545]
                        frame #0 {
                          w537 = FALSE ("Load Actions")
                          n218 = local read "FPGA VI Reference Out"() -> (w544:refnum<k20>)
                          n219 = xnode "Read/Write Control"("FPGA VI Reference In"=w544, "Flush FIFO"=TRUE, "Load Actions Analogue 0"=w537, "Load Actions Analogue 1"=w537, "Load Actions Analogue 2"=w537, "Load Actions Digitals"=w537, "Set Analogue 0"=w537, "Set Analogue 1"=w537, "Set Analogue 2"=w537) -> ("FPGA VI Reference Out"=w542:refnum<k20>)  [unwired: 1 in, 1 out]
                          n220 = xnode "Invoke Method"("FPGA VI Reference In"=w542) -> ("FPGA VI Reference Out"=w541:refnum<k20>)  [unwired: 1 in, 1 out]
                          n221 = xnode "Invoke Method"("FPGA VI Reference In"=w541) -> ("FPGA VI Reference Out"=w540:refnum<k20>)  [unwired: 1 in, 1 out]
                          n222 = xnode "Invoke Method"("FPGA VI Reference In"=w540) -> ("FPGA VI Reference Out"=w539:refnum<k20>)  [unwired: 1 in, 1 out]
                          n223 = xnode "Invoke Method"("FPGA VI Reference In"=w539) -> ("FPGA VI Reference Out"=w538:refnum<k20>)  [unwired: 1 in, 1 out]
                        }
                        frame #1 {
                          n224 = while {
                            tunnel: w545 -> [w546]
                            stop <- w547 stop-if-true
                            # "wait until FPGA target flushes FIFO"
                            n225 = xnode "Read/Write Control"("FPGA VI Reference In"=w546) -> ("Flush FIFO"=w548:bool)  [unwired: 1 in, 2 out]
                            n226 = Not(x=w548) -> (.not. x?=w547:bool)
                          }
                        }
                      }
                    }
                    frame "410" {
                      # "writeDigitals"
                      n227 = TCP Read(connection ID=w557, bytes to read=w554, 7:T5."Buffered" ("mode (standard)"), 9:-1 ("timeout ms (25000)")) -> (connection ID out=w556:refnum<k5>, data out=w551:string)  [unwired: 1 in, 1 out]
                      n228 = local read "FPGA VI Reference Out"() -> (w550:refnum<k20>)
                      n229 = Decimal String To Number(string=w551, default (0L)=u32 0 ("default (0 I32)")) -> (number=w549:u32)  [unwired: 1 in, 1 out]
                      n230 = xnode "Read/Write Control"("FPGA VI Reference In"=w550, "Digitals"=w549) -> ()  [unwired: 1 in, 2 out]
                    }
                    frame "411" {
                      # "writeAnalogue"
                      n231 = TCP Read(connection ID=w572, bytes to read=w568, 7:T5."Buffered" ("mode (standard)"), 9:-1 ("timeout ms (25000)")) -> (connection ID out=w569:refnum<k5>, data out=w574:string, error out=w566:errorcluster)  [unwired: 1 in]
                      n232 = Decimal String To Number(string=w574, default (0L)=u32 0 ("default (0 I32)")) -> (number=w562:u32)  [unwired: 1 in, 1 out]
                      n233 = TCP Read(connection ID=w569, bytes to read=w568, error in (no error)=w566, 7:T5."Buffered" ("mode (standard)"), 9:-1 ("timeout ms (25000)")) -> (connection ID out=w563:refnum<k5>, data out=w564:string)  [unwired: 1 out]
                      n234 = local read "FPGA VI Reference Out"() -> (w559:refnum<k20>)
                      n235 = Decimal String To Number(string=w564, default (0L)=u32 0 ("default (0 I32)")) -> (number=w560:u32)  [unwired: 1 in, 1 out]
                      n236 = case shown="2" w562 {
                        tunnel: w560 -> [w578 w593 w608 w621 w622 w623 _]
                        tunnel: w559 -> [w579 w594 w609 _ _ _ _]
                        frame 0 {
                          n237 = flat-sequence {
                            tunnel: w579 -> [w584]
                            tunnel: w578 -> [w583]
                            tunnel: [w581] -> w577
                            tunnel: [w580] -> w576
                            tunnel: w577 -> [w586]
                            tunnel: w576 -> [w585]
                            frame #0 {
                              n238 = xnode "Read/Write Control"("FPGA VI Reference In"=w584, "Analogue 0"=w583, "Set Analogue 0"=TRUE) -> ("FPGA VI Reference Out"=w581:refnum<k20>, "error out"=w580:errorcluster)  [unwired: 1 in]
                            }
                            frame #1 {
                              n239 = while {
                                tunnel: w586 -> [w590]
                                tunnel: w585 -> [w589]
                                stop <- w587 stop-if-true
                                n240 = xnode "Read/Write Control"("FPGA VI Reference In"=w590, "error in"=w589) -> ("Set Analogue 0"=w588:bool)  [unwired: 2 out]
                                n241 = Not(x=w588) -> (.not. x?=w587:bool)
                              }
                            }
                          }
                        }
                        frame 1 {
                          n242 = flat-sequence {
                            tunnel: w594 -> [w599]
                            tunnel: w593 -> [w598]
                            tunnel: [w596] -> w592
                            tunnel: [w595] -> w591
                            tunnel: w592 -> [w601]
                            tunnel: w591 -> [w600]
                            frame #0 {
                              n243 = xnode "Read/Write Control"("FPGA VI Reference In"=w599, "Analogue 1"=w598, "Set Analogue 1"=TRUE ("Set Analogue 0")) -> ("FPGA VI Reference Out"=w596:refnum<k20>, "error out"=w595:errorcluster)  [unwired: 1 in]
                            }
                            frame #1 {
                              n244 = while {
                                tunnel: w601 -> [w605]
                                tunnel: w600 -> [w604]
                                stop <- w602 stop-if-true
                                n245 = xnode "Read/Write Control"("FPGA VI Reference In"=w605, "error in"=w604) -> ("Set Analogue 1"=w603:bool)  [unwired: 2 out]
                                n246 = Not(x=w603) -> (.not. x?=w602:bool)
                              }
                            }
                          }
                        }
                        frame 2 {
                          n247 = flat-sequence {
                            tunnel: w609 -> [w614]
                            tunnel: w608 -> [w613]
                            tunnel: [w611] -> w607
                            tunnel: [w610] -> w606
                            tunnel: w607 -> [w616]
                            tunnel: w606 -> [w615]
                            frame #0 {
                              n248 = xnode "Read/Write Control"("FPGA VI Reference In"=w614, "Analogue 2"=w613, "Set Analogue 2"=TRUE ("Set Analogue 0")) -> ("FPGA VI Reference Out"=w611:refnum<k20>, "error out"=w610:errorcluster)  [unwired: 1 in]
                            }
                            frame #1 {
                              n249 = while {
                                tunnel: w616 -> [w620]
                                tunnel: w615 -> [w619]
                                stop <- w617 stop-if-true
                                n250 = xnode "Read/Write Control"("FPGA VI Reference In"=w620, "error in"=w619) -> ("Set Analogue 2"=w618:bool)  [unwired: 2 out]
                                n251 = Not(x=w618) -> (.not. x?=w617:bool)
                              }
                            }
                          }
                        }
                        frame 3 {
                          n252 = local write "Analogue Line 3"(w621) -> ()
                        }
                        frame 4 {
                          n253 = local write "Analogue Line 4"(w622) -> ()
                        }
                        frame 5 {
                          n254 = local write "Analogue Line 5"(w623) -> ()
                        }
                        frame Default {
                        }
                      }
                    }
                    frame "413" {
                      # "runSequence"
                    }
                    frame "666", Default {
                    }
                  }
                  "Abort" <- w224
                }
                frame Error {
                }
              }
              n255 = call <vilib>:"General Error Handler.vi"("error in (no error)"=w205, "[exception action] (none:0)"=w207, "[exception code]"=-375003) -> ()  [unwired: 8 in, 5 out]
              n256 = local read "FPGA Status"() -> (w199:string)
              n257 = Bundle(cluster=cluster{"status":string} {"status"="OK"}, "status"=w199) -> (w216:cluster{"status":string})
              n258 = Flatten To JSON "To JSON"(anything=w216) -> (JSON string=w202:string)  [unwired: 2 in, 1 out]
              "ACK sent" <- w202
              n259 = TCP Write(connection ID=w200, data in=w202, error in (no error)=w219) -> (connection ID out=w210:refnum<k5>, error out=w211:errorcluster)  [unwired: 1 in, 1 out]
            }
            "remote address" <- w193
            "remote port" <- w194
          }
          frame Error {
          }
        }
        n260 = local read "Stop VI"() -> (w182:bool)
      }
      n261 = while {
        tunnel: w25 -> [w175]
        tunnel: w26 -> [w174]
        tunnel: "Receive PORT" -> [w173]
        tunnel: w28 -> [w172]
        shift-right: [w153] -> _
        shift-left: _ -> [w152]
        stop <- w166 stop-if-true
        # "Send UDP Update Only when at least one line is changed"
        # "UDP Loop"
        # "Analog 0: Angle\nAnalog 1: Phase\nAnalog 2: Color\nAnalog 3, 4, 5: Laser Power"
        n262 = local read "638 Green Toggle"() -> (w158:bool)
        n263 = local read "488 Blue Toggle"() -> (w160:bool)
        n264 = local read "532 Red Toggle"() -> (w159:bool)
        n265 = Bundle By Name(cluster=T3 {"Digital 0"=FALSE, "Digital 1"=FALSE, "Digital 2"=FALSE}, "Digital 2"=w160, "Digital 1"=w159, "Digital 0"=w158) -> (w157:T3)
        n266 = Cluster To Array(cluster=w157) -> (array=w156:bool[])
        n267 = local read "Analogue Line 1"() -> (w168:u8)
        n268 = local read "Analogue Line 2"() -> (w167:u8)
        n269 = local read "Analogue Line 3"() -> (w165:u32)
        n270 = local read "Analogue Line 4"() -> (w164:u32)
        n271 = local read "Analogue Line 5"() -> (w163:u32)
        n272 = local read "Analogue Line 0"() -> (w169:u8)
        n273 = Boolean Array To Number(Boolean array=w156) -> (number=w162:u32)
        n274 = To Unsigned Byte Integer(number=w162) -> (unsigned 8bit integer=w161:u8)
        n275 = local read "Event"() -> (w170:string)
        n276 = Bundle By Name(cluster=T4 {"Digitals"=0, "Analogue 0"=0, "Analogue 1"=0, "Event"="done", "Analogue 2"=0, "Analogue 3"=0, "Analogue 4"=0, "Analogue 5"=0}, "Digitals"=w161, "Analogue 0"=w169, "Analogue 1"=w168, "Analogue 2"=w167, "Event"=w170, "Analogue 3"=w165, "Analogue 4"=w164, "Analogue 5"=w163) -> (w154:T4)
        n277 = Flatten To JSON(anything=w154) -> (JSON string=w153:string)  [unwired: 2 in, 1 out]
        "UDP Sent" <- w153
        n278 = Not Equal?(x=w153, y=w152) -> (x != y?=w151:bool)
        n279 = Or(x=w151, y=TRUE) -> (x .or. y?=w150:bool)
        n280 = case shown="True" w150 {
          tunnel: w175 -> [_ w181]
          tunnel: w174 -> [_ w179]
          tunnel: w173 -> [_ w178]
          tunnel: w172 -> [_ w177]
          tunnel: w153 -> [_ w176]
          frame False {
          }
          frame True {
            n281 = UDP Write(address=w181, port or service name=w178, connection ID=w179, data in=w176, 8:w177, 9:-1 ("timeout ms (25000)")) -> ()  [unwired: 2 out]
          }
        }
        n282 = local read "Stop VI"() -> (w166:bool)
      }
      n283 = TCP Close Connection(connection ID=w34, error in (no error)=w33) -> (error out=w29:errorcluster)  [unwired: 1 in, 1 out]
      n284 = call <vilib>:"Simple Error Handler.vi"("error in (no error)"=w29) -> ()  [unwired: 4 in, 5 out]
    }
    frame #3 {
      n285 = local read "FPGA VI Reference Out"() -> (w634:refnum<k20>)
      n286 = xnode "Read/Write Control"("FPGA VI Reference In"=w634, "Abort"=TRUE) -> ("FPGA VI Reference Out"=w633:refnum<k20>)  [unwired: 1 in, 1 out]
    }
    frame #4 {
      n287 = xnode "Close FPGA VI Reference"("FPGA VI Reference In"=w635) -> ()  [unwired: 1 in, 1 out]
    }
  }
